vi "Measurement Interval number Writer.vi"(8 "Error In":errorcluster, 10 "Update Time":dbl, 11 "Display Panel.lvlib:Abstract Display.lvclass":refnum<class "Abstract Display.lvclass">) -> (0 "Error Out":errorcluster, 3 "Display Panel.lvlib:Abstract Display.lvclass 2":refnum<class "Abstract Display.lvclass">)   [LabVIEW 2014, in "Display Panel.lvlib" / "Abstract Display.lvclass"]
uses:
  Abstract Display.lvclass
  Abstract Display.lvclass/Abstract Display.ctl
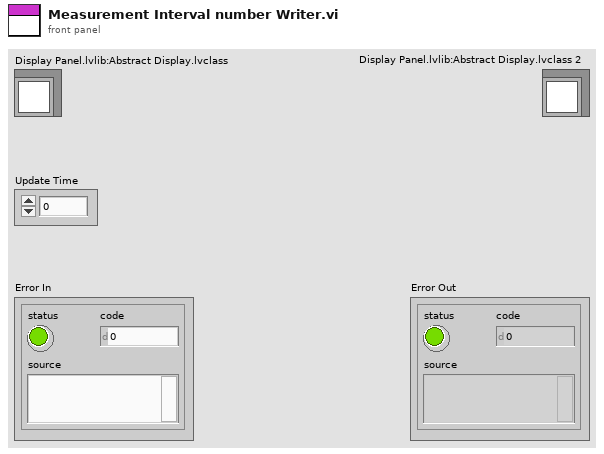
[diagram p1: front panel]
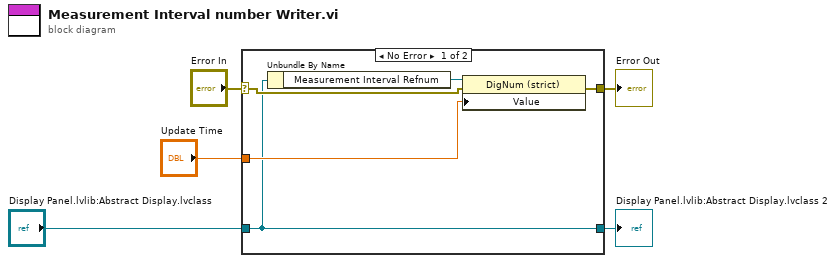
[diagram p0: block diagram]
diagram:
  n1 = case shown="No Error" "Error In" {
    selector: "Error In" -> [w8 w11]
    tunnel: "Display Panel.lvlib:Abstract Display.lvclass" -> [w6 w12]
    tunnel: "Update Time" -> [w9 _]
    tunnel: [w7 w11] -> w2
    tunnel: [w6 w12] -> w1
    frame No Error {
      n2 = Unbundle By Name(w6) -> ("Measurement Interval Refnum"=w10:refnum<vi>)
      n3 = property class="DigNum (strict)"(reference=w10, error in=w8, "Value"=w9) -> (error out=w7:errorcluster)  [unwired: 1 out]
    }
    frame Error {
    }
  }
  "Error Out" <- w2
  "Display Panel.lvlib:Abstract Display.lvclass 2" <- w1
